vi "refresh.vi"(8 "error in":errorcluster, 10 "Engine Configuration":refnum<class "engine configuration.lvclass">, 11 "Shared Memory Editor Node":refnum<class "Shared Memory Editor Node.lvclass">) -> (0 "error out":errorcluster, 2 "Engine Configuration out":refnum<class "engine configuration.lvclass">, 3 "Shared Memory Editor Node Out":refnum<class "Shared Memory Editor Node.lvclass">)   [LabVIEW 2013, in "Shared Memory Editor Node.lvclass"]
doc: "Copyright 2016 National Instruments Corporation\n\nLicensed under the Apache License, Version 2.0 (the \"License\"); you may not use this file except in compliance with the License. You may obtain a copy of the License at http://www.apache.org/licenses/LICENSE-2.0\nUnless required by applicable law or agreed to in writing, software distributed under the License is distributed on an \"AS IS\" BASIS, WITHOUT WARRANTIES OR CONDITIONS OF ANY KIND, either express or implied. See the License for the specific language governing permissions and limitations under the License."
uses:
  Shared Memory Editor Node.lvclass
  <vilib>/NI/Module Execution Interface/Engine Configuration/engine configuration.lvclass
  <vilib>/NI/Configuration Framework/serializable configuration/get alias.vi
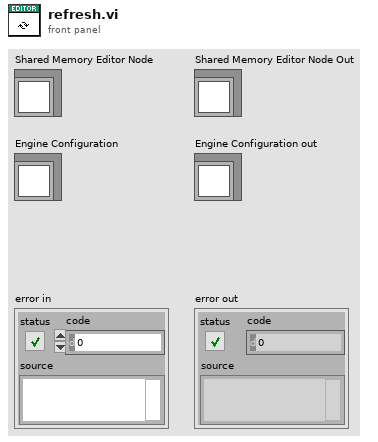
[diagram p1: front panel]
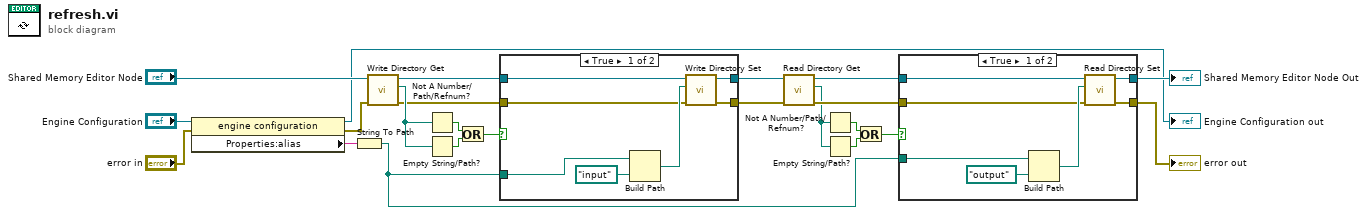
[diagram p0: block diagram]
diagram:
  n1 = property class="engine configuration"(reference="Engine Configuration", error in="error in") -> (reference out=→"Engine Configuration out":refnum<class "engine configuration.lvclass">, error out=w19:errorcluster, "Properties:alias"=w20:string)
  n2 = String To Path(string=w20) -> (path=w5:path)
  n3 = call "Write Directory Get.vi"("error in"=w19, "node"="Shared Memory Editor Node") -> ("error out"=w10:errorcluster, "file directory"=w15:path, "node out"=w11:refnum<class "Shared Memory Editor Node.lvclass">)  [unwired: 7 in]
  n4 = Not A Number/Path/Refnum?(number/path/refnum=w15) -> (NaN/Path/Refnum?=w13:bool)
  n5 = Empty String/Path?(string/path=w15) -> (empty?=w14:bool)
  n6 = Or(x=w13, y=w14) -> (x .or. y?=w12:bool)
  n7 = case shown="True" w12 {
    tunnel: w5 -> [w24 _]
    tunnel: w11 -> [w29 w32]
    tunnel: w10 -> [w27 w31]
    tunnel: [w26 w32] -> w9
    tunnel: [w25 w31] -> w8
    frame True {
      n8 = Build Path(base path=w24, name or relative path=path "input") -> (appended path=w28:path)
      n9 = call "Write Directory Set.vi"("error in"=w27, "file directory"=w28, "node"=w29) -> ("error out"=w25:errorcluster, "node out"=w26:refnum<class "Shared Memory Editor Node.lvclass">)  [unwired: 7 in]
    }
    frame False {
    }
  }
  n10 = call "Read Directory Get.vi"("error in"=w8, "node"=w9) -> ("error out"=w6:errorcluster, "file directory"=w1:path, "node out"=w7:refnum<class "Shared Memory Editor Node.lvclass">)  [unwired: 7 in]
  n11 = Not A Number/Path/Refnum?(number/path/refnum=w1) -> (NaN/Path/Refnum?=w4:bool)
  n12 = Empty String/Path?(string/path=w1) -> (empty?=w3:bool)
  n13 = Or(x=w4, y=w3) -> (x .or. y?=w2:bool)
  n14 = case shown="True" w2 {
    tunnel: w5 -> [w33 _]
    tunnel: w7 -> [w38 w41]
    tunnel: w6 -> [w36 w40]
    tunnel: [w35 w41] -> w22
    tunnel: [w34 w40] -> w21
    frame True {
      n15 = Build Path(base path=w33, name or relative path=path "output") -> (appended path=w37:path)
      n16 = call "Read Directory Set.vi"("error in"=w36, "file directory"=w37, "node"=w38) -> ("error out"=w34:errorcluster, "node out"=w35:refnum<class "Shared Memory Editor Node.lvclass">)  [unwired: 7 in]
    }
    frame False {
    }
  }
  "Shared Memory Editor Node Out" <- w22
  "error out" <- w21
